vi "Teleop.vi"(10 "Match Info":T1={"Autonomous Elapsed Seconds"=0.0, "TeleOp Elapsed Seconds"=0.0, "Disabled Elapsed Seconds"=0.0, "Visited Autonomous"=FALSE, "Visited TeleOp"=FALSE, "Visited Disabled"=FALSE, "Autonomous Settings"={"Autonomous Style"=enum."Independent", "VI Refnum"=refnum}}, 11 "Call Context":T2) -> ()   [LabVIEW 2017]
doc: "This VI is called for each enabled TeleOp packet received from the DS. It is typically used to read from joysticks and other inputs and update I/O or setpoints for timed control loops. It should complete and return within 20 milliseconds or risk missing DS packets."
uses:
  <vilib>/Rock Robotics/WPI/DriverStation/WPI_DriverStationDerivedRobotMode.ctl
  <vilib>/Rock Robotics/WPI/DriverStation/WPI_DriverStationMatch Info.ctl
  <vilib>/Rock Robotics/WPI/Utilities/WPI_GetSetVariantRefNum.vi
  <vilib>/Rock Robotics/Network Tables/NT Write Boolean Array.vi
  <vilib>/Rock Robotics/Network Tables/NT Write Numeric Array.vi
  Framework/Robot Global Data.vi
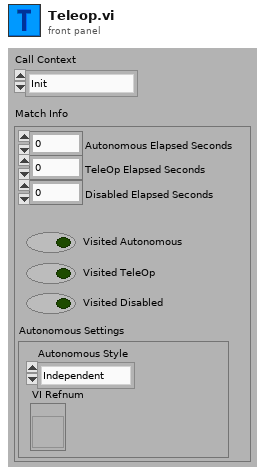
[diagram p1: front panel]
types:
  T1 = typedef "WPI_DriverStationMatch Info.ctl" = cluster{"Autonomous Elapsed Seconds":dbl, "TeleOp Elapsed Seconds":dbl, "Disabled Elapsed Seconds":dbl, "Visited Autonomous":bool, "Visited TeleOp":bool, "Visited Disabled":bool, "Autonomous Settings":cluster{"Autonomous Style":enum16{"Iterative", "Independent"}, "VI Refnum":refnum<vi>}}
  T2 = typedef "WPI_DriverStationDerivedRobotMode.ctl" = enum16{"Init", "Execute", "Stop"}
  T3 = typedef "WPI_JoystickDevRef.ctl" = cluster{"Device":T4}
  T4 = typedef "WPI_JoystickDeviceEnum.ctl" = enum16{"USB 0", "USB 1", "USB 2", "USB 3", "USB 4", "USB 5"}
  T5 = typedef "Command Status Info.ctl" = cluster{"Name":string, "Status":T6, "notifier out":T7}
  T6 = typedef "Completion Status.ctl" = enum16{"Successful", "Aborted", "Incomplete"}
  T7 = typedef "Completion Notifier.ctl" = refnum<notifier>
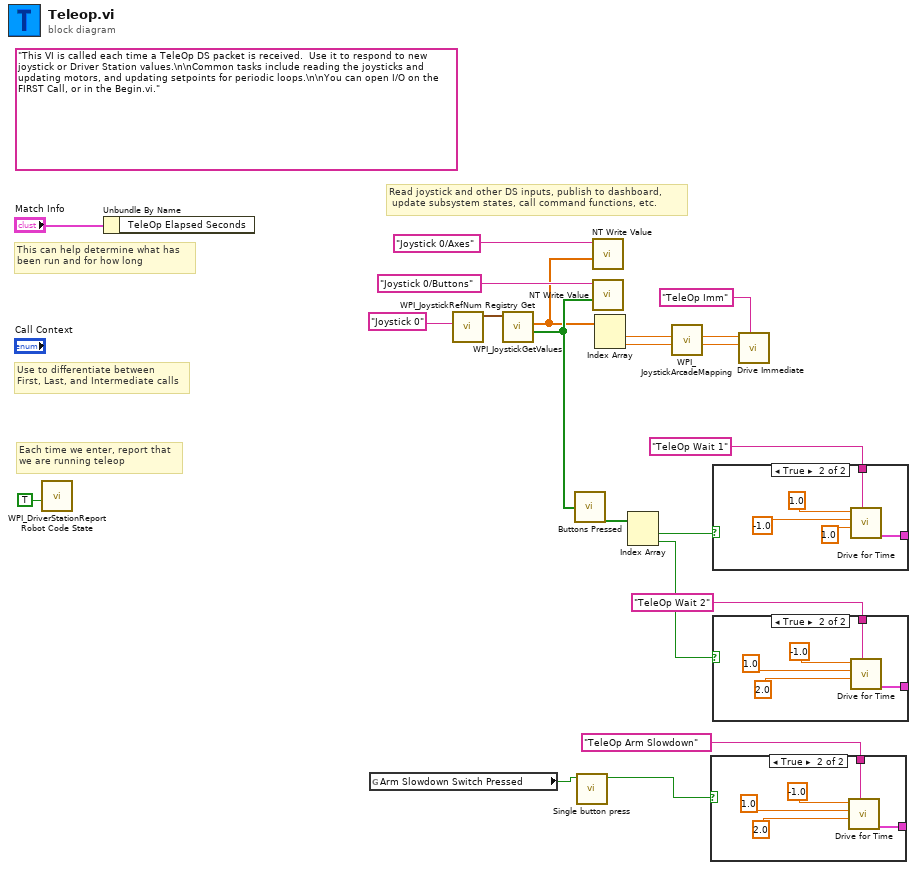
[diagram p0: block diagram]
diagram:
  (unwired) "This VI is called each time a TeleOp DS packet is received.  Use it to respond to new joystick or Driver Station values.\n\nCommon tasks include reading the joysticks and updating motors, and updating setpoints for periodic loops.\n\nYou can open I/O on the FIRST Call, or in the Begin.vi."
  # "Read joystick and other DS inputs, publish to dashboard,\n update subsystem states, call command functions, etc."
  # "Each time we enter, report that\nwe are running teleop"
  # "Use to differentiate between\nFirst, Last, and Intermediate calls"
  # "This can help determine what has\nbeen run and for how long"
  n1 = call <vilib>:"WPI_DriverStationReport Robot Code State.vi"("TeleOp"=TRUE ("Autonomous")) -> ()  [unwired: 10 in, 1 out]
  n2 = Unbundle By Name("Match Info") -> ()  [unwired: 1 out]
  n3 = global read "Robot Global Data.vi" "Arm Slowdown Switch Pressed"() -> (w2:bool)
  n4 = call <vilib>:"WPI_JoystickRefNum Registry Get.vi"("refnum name"="Joystick 0") -> ("JoystickDevRef"=w18:T3)  [unwired: 1 in, 9 out]
  n5 = call <vilib>:"WPI_JoystickGetValues.vi"("JoystickDevRef"=w18) -> ("Buttons"=w6:bool[], "Axes"=w5:dbl[])  [unwired: 6 in, 3 out]
  n6 = call "Buttons Pressed.vi"("Button Values"=w6) -> ("Button Presses"=w14:bool[])
  n7 = call "Single button press.vi"("Button Value"=w2) -> ("Button Press"=w1:bool)  [unwired: 10 in]
  n8 = call-poly <vilib>:"NT Write Value.vi"("Numeric Array"=w5, "Name"="Joystick 0/Axes") -> ()  [unwired: 9 in, 1 out]
  n9 = call-poly <vilib>:"NT Write Value.vi"("Boolean Array"=w6, "Name"="Joystick 0/Buttons") -> ()  [unwired: 9 in, 1 out]
  n10 = Index Array(array=w5) -> (element #1=w9:dbl, element #2=w8:dbl)  [unwired: 2 in]
  n11 = Index Array(array=w14) -> (element #1=w13:bool, element #2=w12:bool)  [unwired: 2 in]
  n12 = call <vilib>:"WPI_JoystickArcadeMapping.vi"("Y axis value"=w8, "X axis value"=w9) -> ("Right Motor Value"=w10:dbl, "Left Motor Value"=w11:dbl)  [unwired: 8 in]
  n13 = case shown="True" w1 {
    tunnel: [_ w24] -> _
    tunnel: "TeleOp Arm Slowdown" ("Description") -> [_ w23]
    frame False {
    }
    frame True {
      n14 = call "Drive for Time.vi"("Description"=w23, "Seconds"=2.0, "Right Speed"=1.0, "Left Speed"=-1.0) -> ("Command Info Out"=w24:T5)  [unwired: 6 in, 1 out]
    }
  }
  n15 = case shown="True" w13 {
    tunnel: [_ w30] -> _
    tunnel: "TeleOp Wait 1" ("Description") -> [_ w29]
    frame False {
    }
    frame True {
      n16 = call "Drive for Time.vi"("Description"=w29, "Seconds"=1.0, "Right Speed"=-1.0, "Left Speed"=1.0) -> ("Command Info Out"=w30:T5)  [unwired: 6 in, 1 out]
    }
  }
  n17 = case shown="True" w12 {
    tunnel: [_ w34] -> _
    tunnel: "TeleOp Wait 2" ("Description") -> [_ w33]
    frame False {
    }
    frame True {
      n18 = call "Drive for Time.vi"("Description"=w33, "Seconds"=2.0, "Right Speed"=1.0, "Left Speed"=-1.0) -> ("Command Info Out"=w34:T5)  [unwired: 6 in, 1 out]
    }
  }
  n19 = call "Drive Immediate.vi"("Description"="TeleOp Imm", "Right Setpoint"=w10, "Left Setpoint"=w11) -> ()  [unwired: 8 in, 1 out]
